vi "Test List All Categories.vi"(8 "error in (no error)":errorcluster) -> (0 "error out":errorcluster)   [LabVIEW 2013, in "JKI State Machine API - Tests.lvlib"]
uses:
  JKI State Machine API - Tests.lvlib
  <vilib>/addons/_JKI Toolkits/Caraya/classes/Assert/Assert.lvclass
  <vilib>/addons/_JKI Toolkits/Caraya/classes/Test/Test.lvclass
  source/JKI SM/JKI SM.lvclass
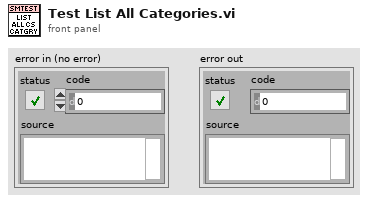
[diagram p1: front panel]
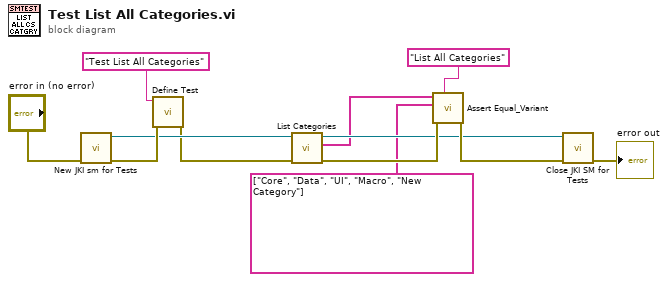
[diagram p0: block diagram]
diagram:
  n1 = call "New JKI sm for Tests.vi"("error in (no error)"="error in (no error)") -> ("error out"=w12:errorcluster, "JKI SM out"=w6:refnum<class "JKI SM.lvclass">)  [unwired: 9 in]
  n2 = call <vilib>:"Define Test.vi"("error in (no error)"=w12, "Label (VI Title)"="Test List All Categories") -> ("error out"=w4:errorcluster)  [unwired: 9 in]
  n3 = call "List Categories.vi"("error in (no error)"=w4, "JKI SM in"=w6) -> ("error out"=w5:errorcluster, "All State Categories"=w2:string[], "JKI SM out"=w3:refnum<class "JKI SM.lvclass">)  [unwired: 6 in, 1 out]
  n4 = call <vilib>:"Assert Equal_Variant.vi"("Label"="List All Categories", "error in (no error)"=w5, "Y"=string[] ["Core", "Data", "UI", "Macro", "New Category"] ("All State Categories"), "X"=w2) -> ("error out"=w9:errorcluster)  [unwired: 7 in]
  n5 = call "Close JKI SM for Tests.vi"("error in (no error)"=w9, "JKI SM in"=w3) -> ("error out"=→"error out":errorcluster)  [unwired: 9 in]
